vi "XNETDB.Add.vi"(8 "error in (no error)":errorcluster, 11 "Databases Section Ref":T1 format="%.0x") -> (0 "error out":errorcluster)   [LabVIEW 2015, in "Diagnostics Addon System Explorer.lvlib"]
uses:
  Diagnostics Addon System Explorer.lvlib
  <vilib>/NI Veristand/Custom Device API/Custom Device Item Ref.ctl
  <vilib>/NI Veristand/Custom Device API/Set Item Property (String).vi
  Shared/SubVIs/Constants.vi
  Shared/Diagnostics Addon Shared.lvlib
  <vilib>/NI Veristand/Custom Device API/Custom Device API.lvlib
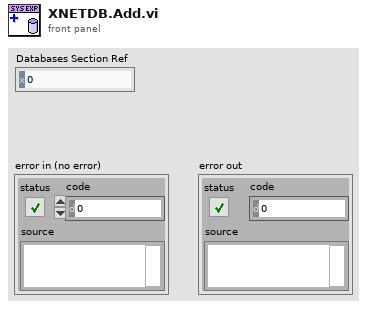
[diagram p1: front panel]
types:
  T1 = typedef "Custom Device API.lvlib/Custom Device Item Ref.ctl" = u64
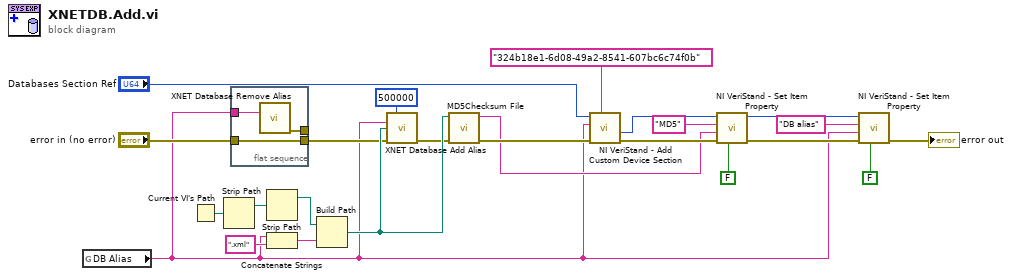
[diagram p0: block diagram]
diagram:
  n1 = global read "Constants.vi" "DB Alias"() -> (w1:string)
  n2 = Current VI's Path() -> (path=w18:path)
  n3 = Strip Path(path=w18) -> (stripped path=w22:path)  [unwired: 1 out]
  n4 = flat-sequence {
    tunnel: [w27] -> w3
    tunnel: "error in (no error)" -> [w27]
    tunnel: [w26] -> _
    tunnel: w1 -> [w25]
    frame #0 {
      n5 = call <vilib>:"XNET Database Remove Alias.vi"("alias"=w25) -> ("error out"=w26:errorcluster)  [unwired: 14 in]
    }
  }
  n6 = Strip Path(path=w22) -> (stripped path=w17:path)  [unwired: 1 out]
  n7 = Concatenate Strings(w1, ".xml" ("string")) -> (w20:string)
  n8 = Build Path(base path=w17, name or relative path=w20) -> (appended path=w16:path)
  n9 = call <vilib>:"XNET Database Add Alias.vi"("default baud rate (0)"=u32 500000, "alias"=w1, "filepath"=w16, "error in (no error)"=w3) -> ("error out"=w15:errorcluster)  [unwired: 11 in]
  n10 = call <vilib>:"MD5Checksum File.vi"("error in (no error)"=w15, "Path"=w16) -> ("error out"=w5:errorcluster, "MD5 message-digest"=w4:string)  [unwired: 8 in]
  n11 = call <vilib>:"NI VeriStand - Add Custom Device Section.vi"("GUID (Default Section)"="324b18e1-6d08-49a2-8541-607bc6c74f0b", "error in (no error)"=w5, "Section Name"=w1, "Parent Ref in"="Databases Section Ref") -> ("error out"=w11:errorcluster, "Section Ptr"=w12:T1)  [unwired: 4 in, 2 out]
  n12 = call-poly <vilib>:"NI VeriStand - Set Item Property.vi"("Binary String (T)"=FALSE, "error in (no error)"=w11, "Value"=w4, "Property Name"="MD5", "Item Ref in"=w12) -> ("error out"=w10:errorcluster, "Item Ref out"=w9:T1)  [unwired: 4 in, 1 out]
  n13 = call-poly <vilib>:"NI VeriStand - Set Item Property.vi"("Binary String (T)"=FALSE, "error in (no error)"=w10, "Value"=w1, "Property Name"="DB alias", "Item Ref in"=w9) -> ("error out"=→"error out":errorcluster)  [unwired: 4 in, 2 out]
